vi "Shooter Controller.vi"(8 "error in":errorcluster) -> ()   [LabVIEW 2020]
doc: "This VI executes continuously carrying out the current operation and responding to updates or new operations. It will often contain the timing or control code that is difficult to place directly in TeleOp. This VI generally opens all sensors and motors and isolates the rest of the robot code from knowing how the operations are carried out."
uses:
  <vilib>/Rock Robotics/WPI/Framework/Completion Status.ctl
  Shooter Setpoints.ctl
  Shooter Operations.ctl
  <vilib>/Rock Robotics/WPI/SafetyOutput/WPI_SafetyOutputConfigMenu.ctl
  <vilib>/Rock Robotics/WPI/ThirdParty/REV Robotics/REVLib/Typedef/Spark MAX Motor Type.ctl
  <vilib>/Rock Robotics/WPI/ThirdParty/REV Robotics/REVLib/Typedef/Spark MAX Idle Mode.ctl
  <vilib>/Rock Robotics/Network Tables/NT Write Number.vi
panel:
  in  "Interactive Values":T1
  out "Current\nCmd":string
  in  "Buttons":cluster{"Execute Cmd":bool, "Abort Cmd":bool}
  out "Command Timing":cluster{"Start Time (ms)":u32, "Iterations":i32}
  out "Status":T3
  # "Tip: It may be helpful to observe inputs and sensor values.\nYou may also want to display tuning or debugging controls."
  # "Interactive Command: You may fill in the settings for a command\nand schedule it with the Execute button. You can observe and abort\nany command while fine tuning the code for the controller."
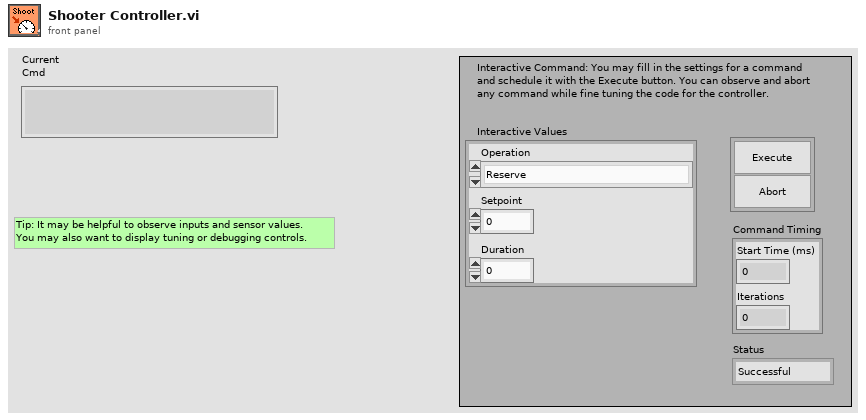
[diagram p1: front panel]
types:
  T1 = typedef "Shooter Setpoints.ctl" = cluster{"Operation":T2, "Setpoint":dbl, "Duration":dbl}
  T2 = typedef "Shooter Operations.ctl" = enum16{"Reserve", "Read Current", "Immediate", "for Time"}
  T3 = typedef "Completion Status.ctl" = enum16{"Successful", "Aborted", "Incomplete"}
  T4 = typedef "Spark MAX Idle Mode.ctl" = enum16{"Coast", "Brake"}
  T5 = typedef "Spark MAX Motor Type.ctl" = enum16{"Brushed", "Brushless"}
  T6 = typedef "WPI_SafetyOutputConfigMenu.ctl" = enum16{"Enable", "Disable"}
  T7 = typedef "WPI_MotorControlDeviceRef.ctl" = cluster{"DeviceStatus":errorcluster, "Type":T8, "PWM":cluster{"PWM Channel":T9, "DeadBand":T10}, "CAN":cluster{"Device Number":u8, "SetOutput VI Ref":variant, "GetOutput VI Ref":variant, "Enable VI Ref":variant, "Disable VI Ref":variant, "Data":variant}, "Invert":bool, "DIO PWM":cluster{"PWM \"Enable\" Channel":T9, "DIOChannel":T11, "PWM Rate":dbl}}
  T8 = typedef "WPI_MotorControlType.ctl" = enum16{"PWM", "CAN", "DIO PWM"}
  T9 = typedef "FPGA_DIOPWMChannel.ctl" = enum8{"PWM 0", "PWM 1", "PWM 2", "PWM 3", "PWM 4", "PWM 5", "PWM 6", "PWM 7", "PWM 8", "PWM 9", "PWM MXP 0", "PWM MXP 1", "PWM MXP 2", "PWM MXP 3", "PWM MXP 4", "PWM MXP 5", "PWM MXP 6", "PWM MXP 7", "PWM MXP 8", "PWM MXP 9", "Invalid"}
  T10 = typedef "WPI_PWMDeadband.ctl" = cluster{"Name":string, "maxPositivePwm":i32, "minPositivePwm":i32, "centerPwm":i32, "maxNegativePwm":i32, "minNegativePwm":i32, "angularRange":u16}
  T11 = typedef "FPGA_DIOChannel.ctl" = enum8{"DIO 0", "DIO 1", "DIO 2", "DIO 3", "DIO 4", "DIO 5", "DIO 6", "DIO 7", "DIO 8", "DIO 9", "DIO MXP 0", "DIO MXP 1", "DIO MXP 2", "DIO MXP 3", "DIO MXP 4", "DIO MXP 5", "DIO MXP 6", "DIO MXP 7", "DIO MXP 8", "DIO MXP 9", "DIO MXP 10", "DIO MXP 11", "DIO MXP 12", "DIO MXP 13", "DIO MXP 14", "DIO MXP 15", "SPI Port CS1", "SPI Port CS2", "SPI Port CS3", "SPI Port MISO", "SPI Port MOSI", "Invalid"}
  T12 = typedef "Command Status Info.ctl" = cluster{"Name":string, "Status":T3, "notifier out":T13}
  T13 = typedef "Completion Notifier.ctl" = refnum<notifier>
  T14 = cluster{"Current Command":T1, "Command Timing":cluster{"Start Time (ms)":u32, "Iterations":i32}, "Command Arguments":cluster{"Command Info":T12, "Description":string, "Default Command":T1, "queue out":refnum<queue>, "Subsystem Name":string}}
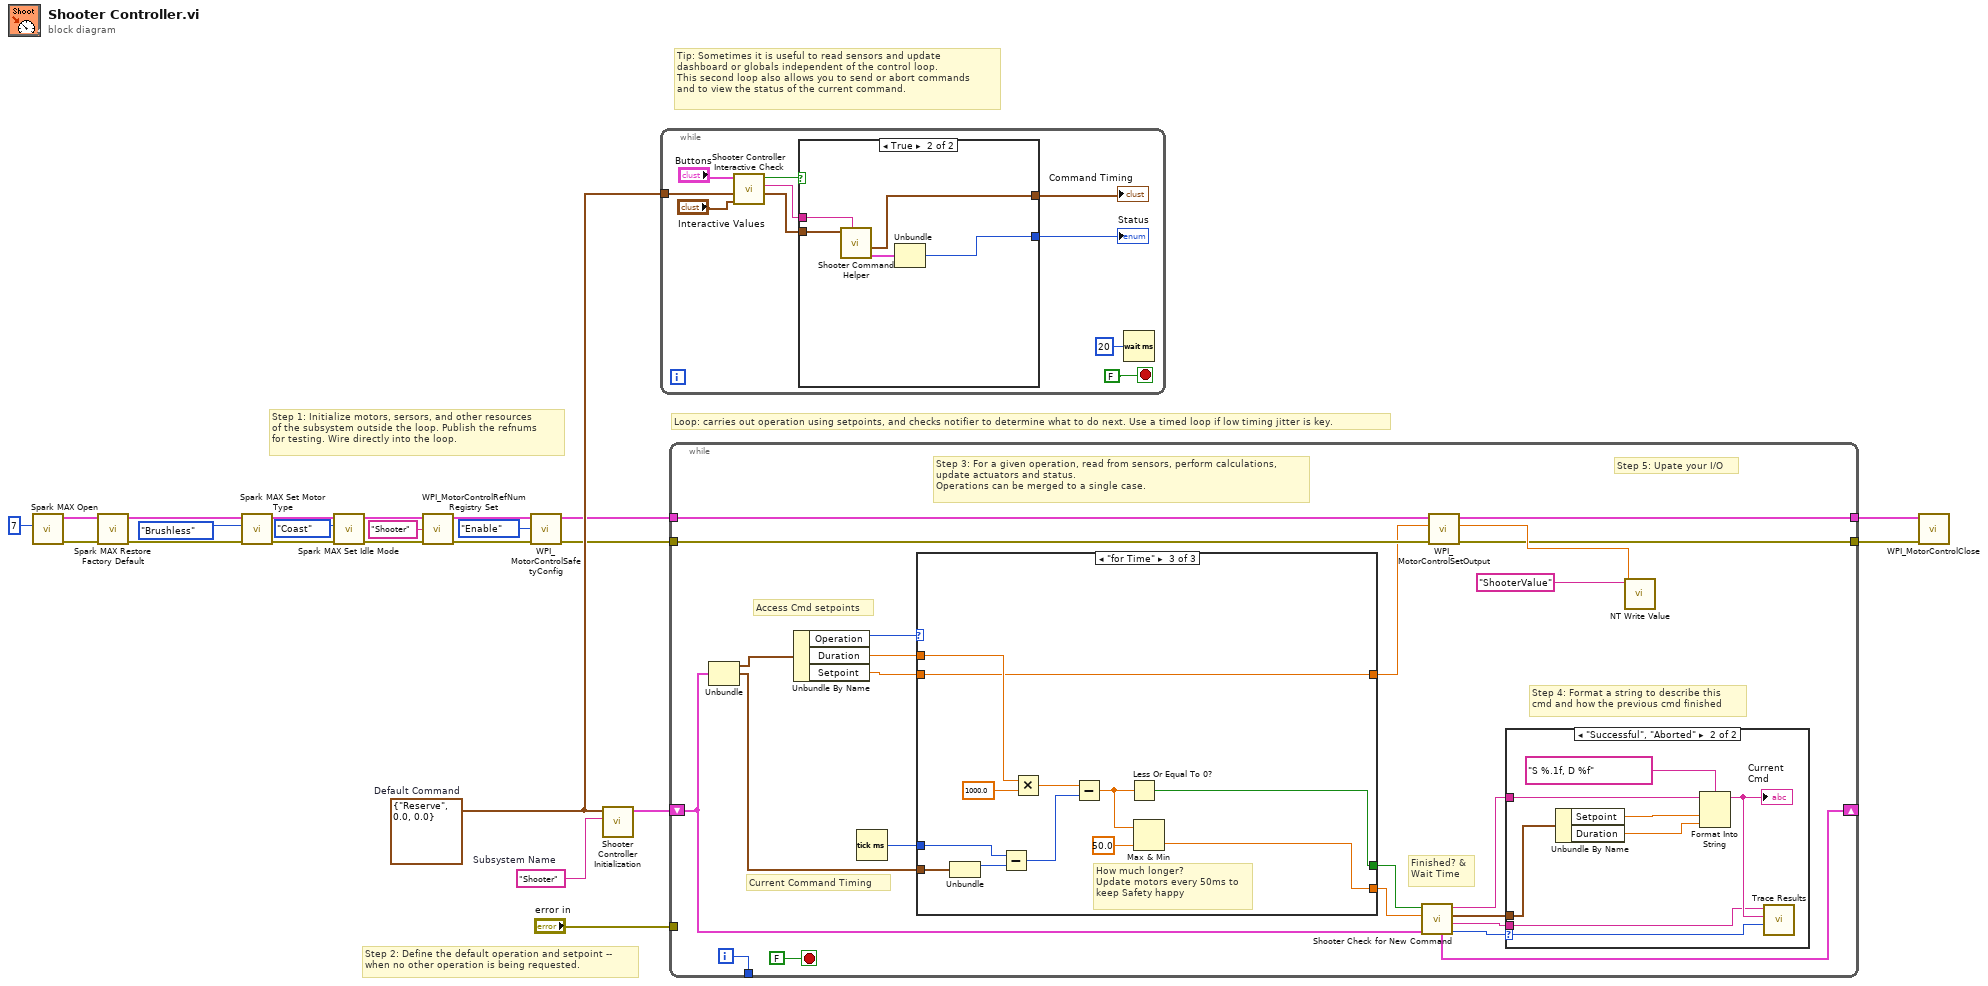
[diagram p0: block diagram]
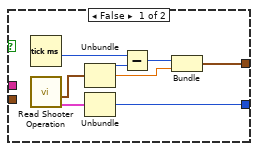
[diagram p2: hidden frame]
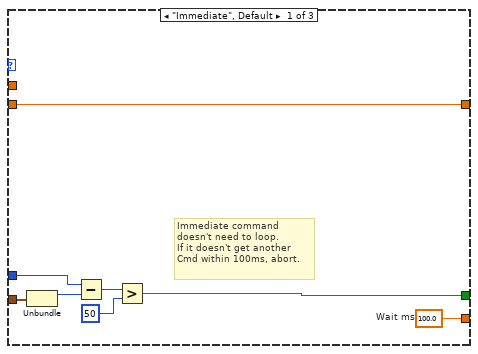
[diagram p4: hidden frame]
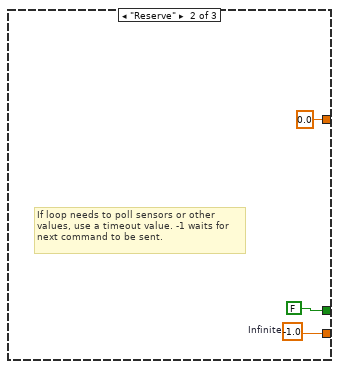
[diagram p5: hidden frame]
diagram:
  w20 = T1 {"Operation"=enum."Reserve", "Setpoint"=0.0, "Duration"=0.0}  # Default Command
  w21 = "Shooter"  # Subsystem Name
  # "Tip: Sometimes it is useful to read sensors and update\ndashboard or globals independent of the control loop.\nThis second loop also allows you to send or abort commands\nand to view the status of the current command."
  # "Step 2: Define the default operation and setpoint --\nwhen no other operation is being requested."
  # "Step 1: Initialize motors, sersors, and other resources\nof the subsystem outside the loop. Publish the refnums\nfor testing. Wire directly into the loop."
  # "Loop: carries out operation using setpoints, and checks notifier to determine what to do next. Use a timed loop if low timing jitter is key."
  n1 = call <vilib>:"Spark MAX Open.vi"("Device Number"=u8 7) -> ("error out"=w19:errorcluster, "MotorControlDeviceRef"=w18:T7)  [unwired: 9 in]
  n2 = call <vilib>:"Spark MAX Restore Factory Default.vi"("error in"=w19, "MotorControlDeviceRef"=w18) -> ("error out"=w4:errorcluster, "MotorControlDeviceRef"=w6:T7)  [unwired: 8 in]
  n3 = call <vilib>:"Spark MAX Set Motor Type.vi"("error in (no error)"=w4, "Motor Type"=Spark_MAX_Motor_Type."Brushless", "MotorControlDevRef"=w6) -> ("error out"=w3:errorcluster, "MotorControlDeviceRef"=w5:T7)  [unwired: 7 in]
  n4 = call <vilib>:"Spark MAX Set Idle Mode.vi"("error in (no error)"=w3, "Idle Mode"=Spark_MAX_Idle_Mode."Coast", "MotorControlDeviceRef in"=w5) -> ("error out"=w2:errorcluster, "MotorControlDeviceRef out"=w1:T7)  [unwired: 7 in]
  n5 = call <vilib>:"WPI_MotorControlRefNum Registry Set.vi"("error in (no error)"=w2, "refnum name"="Shooter", "MotorControlDevRef"=w1) -> ("error out"=w17:errorcluster, "MotorControlDevRef"=w16:T7)  [unwired: 7 in]
  n6 = call <vilib>:"WPI_MotorControlSafetyConfig.vi"("error in (no error)"=w17, "mode"=WPI_SafetyOutputConfigMenu."Enable", "MotorControlDevRef"=w16) -> ("error out"=w12:errorcluster, "MotorControlDevRef"=w13:T7)  [unwired: 7 in]
  n7 = call "Shooter Controller Initialization.vi"("Subsystem Name"=w21, "Default Command"=w20) -> ("Current Command"=w22:T14)  [unwired: 9 in]
  n8 = while {
    tunnel: w20 -> [w30]
    stop <- FALSE stop-if-true
    n9 = call "Shooter Controller Interactive Check.vi"("Interactive Command in"="Interactive Values", "Default Command"=w30, "Buttons"="Buttons") -> ("Interactive Command out"=w27:T1, "Trace String"=w28:string, "Schedule"=w29:bool)  [unwired: 6 in]
    n10 = case shown="True" w29 {
      tunnel: [w41 w46] -> w26
      tunnel: w27 -> [_ w44]
      tunnel: [w37 w42] -> w25
      tunnel: w28 -> [_ w45]
      frame False {
        n11 = Tick Count (ms)() -> (millisecond timer value=w36:u32)
        n12 = call "Read Shooter Operation.vi"() -> ("Command Info"=w34:T12, "SubSystem Data"=w35:T1)  [unwired: 9 in, 1 out]
        n13 = Unbundle(w35) -> ("Operation"=w40:T2, "Setpoint"=w38:dbl)  [unwired: 1 out]
        n14 = Unbundle(w34) -> ("Status"=w41:T3)  [unwired: 2 out]
        n15 = Subtract(x=w36, y=w40) -> (x-y=w39:u32)
        n16 = Bundle(w39, "Setpoint"=w38) -> (w37:cluster{u32, "Setpoint":dbl})  [unwired: 1 in]
      }
      frame True {
        n17 = call "Shooter Command Helper.vi"("Description"=w45, "SubSystem Data"=w44) -> ("Command Info Out"=w43:T12, "Command Timing"=w42:cluster{"Start Time (ms)":u32, "Iterations":i32})  [unwired: 7 in, 1 out]
        n18 = Unbundle(w43) -> ("Status"=w46:T3)  [unwired: 2 out]
      }
    }
    "Status" <- w26
    "Command Timing" <- w25
    n19 = Wait (ms)(milliseconds to wait=u32 20) -> ()  [unwired: 1 out]
  }
  n20 = while {
    shift-right: [w61] -> _
    shift-left: w22 -> [w54]
    tunnel: [w68] -> _
    tunnel: "error in" -> [_]
    tunnel: w13 -> [w53]
    tunnel: w12 -> [w52]
    tunnel: [w48] -> w10
    tunnel: [w47] -> w9
    i -> [w68]
    stop <- FALSE stop-if-true
    # "Step 5: Upate your I/O"
    # "Step 4: Format a string to describe this\ncmd and how the previous cmd finished"
    # "Current Command Timing"
    # "Access Cmd setpoints"
    # "Finished? &\nWait Time"
    # "Step 3: For a given operation, read from sensors, perform calculations,\nupdate actuators and status.\nOperations can be merged to a single case."
    n21 = Unbundle(w54) -> ("Current Command"=w67:T1, "Command Timing"=w63:cluster{"Start Time (ms)":u32, "Iterations":i32})  [unwired: 1 out]
    n22 = Unbundle By Name(w67) -> ("Operation"=w66:T2, "Duration"=w65:dbl, "Setpoint"=w62:dbl)
    n23 = Tick Count (ms)() -> (millisecond timer value=w64:u32)
    n24 = case shown="\"for Time\"" w66 {
      tunnel: [w85 w88 w91] -> w59
      tunnel: [w79 FALSE ("ignore previous (F)") w92] -> w60
      tunnel: w63 -> [w81 _ w93]
      tunnel: w65 -> [_ _ w90]
      tunnel: w64 -> [w80 _ w94]
      tunnel: w62 -> [w78 _ w89]
      tunnel: [w78 0.0 ("Setpoint") w89] -> w51
      frame "Immediate", Default {
        w85 = 100.0  # Wait ms
        # "Immediate command\ndoesn't need to loop.\nIf it doesn't get another\nCmd within 100ms, abort."
        n25 = Unbundle(w81) -> ("Start Time (ms)"=w84:u32)  [unwired: 1 out]
        n26 = Subtract(x=w80, y=w84) -> (x-y=w83:u32)
        n27 = Greater?(x=w83, y=u8 50 ("Left Motor")) -> (0:w79:bool)
      }
      frame "Reserve" {
        w88 = -1.0  # Infinite
        # "If loop needs to poll sensors or other\nvalues, use a timeout value. -1 waits for\nnext command to be sent."
      }
      frame "for Time" {
        # "How much longer?\nUpdate motors every 50ms to\nkeep Safety happy"
        n28 = Unbundle(w93) -> ("Start Time (ms)"=w99:u32)  [unwired: 1 out]
        n29 = Subtract(x=w94, y=w99) -> (x-y=w97:u32)
        n30 = Multiply(x=w90, y=1000.0) -> (x*y=w98:dbl)
        n31 = Subtract(x=w98, y=w97) -> (x-y=w100:dbl)
        n32 = Less Or Equal To 0?(x=w100) -> (x <= 0?=w92:bool)
        n33 = Max & Min(x=w100, y=50.0) -> (min(x,y)=w91:dbl)  [unwired: 1 out]
      }
    }
    n34 = call "Shooter Check for New Command.vi"("Current Command"=w54, "Wait time (ms)"=w59, "Finished?"=w60) -> ("Completion"=w55:T3, "Subsystem Name"=w56:string, "Current Command"=w57:T1, "Initial Trace String"=w58:string, "NextCommand"=w61:T14)  [unwired: 4 in]
    n35 = call <vilib>:"WPI_MotorControlSetOutput.vi"("error in (no error)"=w52, "Output"=w51, "MotorControlDevRef"=w53) -> ("error out"=w47:errorcluster, "Motor Output"=w50:dbl, "MotorControlDevRef"=w48:T7)  [unwired: 6 in]
    n36 = case shown="\"Successful\", \"Aborted\"" w55 {
      selector: w55 -> [_ w77]
      tunnel: w58 -> [_ w73]
      tunnel: w57 -> [_ w74]
      tunnel: w56 -> [_ w70]
      frame "Incomplete", Default {
        # "Continuing current command"
      }
      frame "Successful", "Aborted" {
        # "Report and setup for next command"
        n37 = Unbundle By Name(w74) -> ("Setpoint"=w76:dbl, "Duration"=w71:dbl)
        n38 = Format Into String(format string="S %.1f, D %f", initial string=w73, w76, w71) -> (resulting string=w72:string)  [unwired: 1 in, 1 out]
        "Current\nCmd" <- w72
        n39 = call <vilib>:"Trace Results.vi"("Status of previous command"=w77, "Description"=w72, "Subsystem"=w70) -> ()  [unwired: 9 in]
      }
    }
    n40 = call-poly <vilib>:"NT Write Value.vi"("Numeric"=w50, "Name"="ShooterValue") -> ()  [unwired: 9 in, 1 out]
  }
  n41 = call <vilib>:"WPI_MotorControlClose.vi"("error in"=w9, "MotorControlDevRef"=w10) -> ()  [unwired: 9 in, 1 out]
